vi "VCL_2_TSV.vi"(8 "error in (no error)":errorcluster, 11 "Path to VCL file":path) -> (0 "error out":errorcluster, 1 "standard output":string, 3 "path to txt file":path)   [LabVIEW 2019, in "VCL_2_DSC.lvclass"]
uses:
  VCL_2_DSC.lvclass
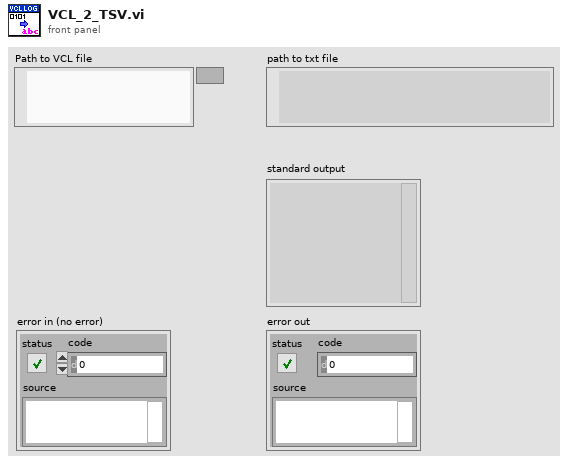
[diagram p1: front panel]
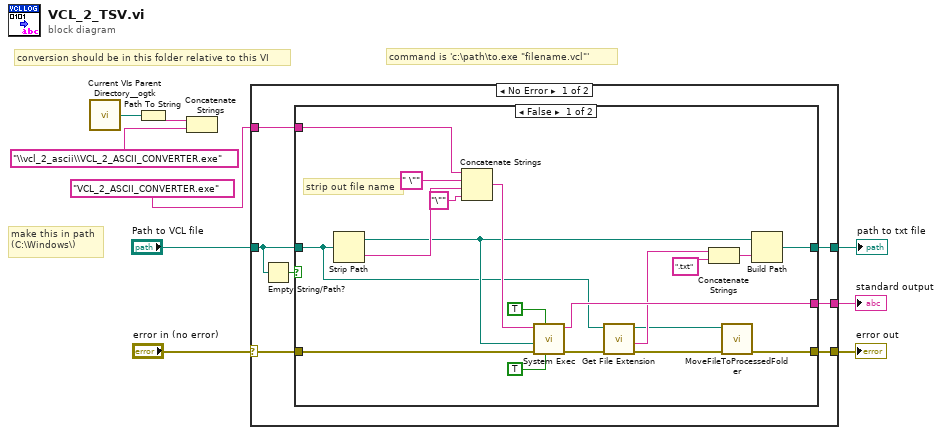
[diagram p0: block diagram]
diagram:
  # "make this in path\n(C:\\Windows\\)"
  # "command is 'c:\\path\\to.exe \"filename.vcl\"'"
  # "conversion should be in this folder relative to this VI"
  n1 = call <userlib>:"Current VIs Parent Directory__ogtk.vi"() -> ("Parent Directory (+ Relative)"=w7:path)  [unwired: 5 in]
  n2 = Path To String(path=w7) -> (string=w6:string)
  n3 = Concatenate Strings(w6, "\\vcl_2_ascii\\VCL_2_ASCII_CONVERTER.exe" ("full path to VCL_2_ASCII_CONVERTER.exe")) -> ()  [unwired: 1 out]
  n4 = case shown="No Error" "error in (no error)" {
    selector: "error in (no error)" -> [w11 w37]
    tunnel: [w16 w37] -> w9
    tunnel: [w15 _] -> w8
    tunnel: "VCL_2_ASCII_CONVERTER.exe" ("full path to VCL_2_ASCII_CONVERTER.exe") -> [w14 _]
    tunnel: "Path to VCL file" -> [w12 _]
    tunnel: [w10 _] -> w2
    frame No Error {
      n5 = Empty String/Path?(string/path=w12) -> (empty?=w13:bool)
      n6 = case shown="False" w13 {
        tunnel: w11 -> [w35 w36]
        tunnel: [w20 w36] -> w16
        tunnel: [w30 _] -> w15
        tunnel: w12 -> [w17 _]
        tunnel: w14 -> [w29 _]
        tunnel: [w23 _] -> w10
        frame False {
          # "strip out file name"
          n7 = Strip Path(path=w17) -> (stripped path=w18:path, name=w32:string)
          n8 = Concatenate Strings(w29, " \"" ("string"), w32, "\"" ("string")) -> (w33:string)
          n9 = call <vilib>:"System Exec.vi"("run minimized? (F)"=TRUE, "wait until completion? (T)"=TRUE, "error in (no error)"=w35, "working directory"=w18, "command line"=w33) -> ("error out"=w19:errorcluster, "standard output"=w30:string)  [unwired: 3 in, 2 out]
          n10 = call <vilib>:"Get File Extension.vi"("error in (no error)"=w19, "file"=w17) -> ("error out"=w21:errorcluster, "filename without extension"=w25:string, "dup file"=w22:path)  [unwired: 5 in, 2 out]
          n11 = Concatenate Strings(w25, ".txt" ("pattern")) -> (w24:string)
          n12 = call "MoveFileToProcessedFolder.vi"("error in (no error)"=w21, "source file"=w22) -> ("error out"=w20:errorcluster)  [unwired: 8 in, 1 out]
          n13 = Build Path(base path=w18, name or relative path=w24) -> (appended path=w23:path)
        }
        frame True {
        }
      }
    }
    frame Error {
    }
  }
  "standard output" <- w8
  "error out" <- w9
  "path to txt file" <- w2
